vi "get Data.vi"(11 "IO in":refnum<class "IO.lvclass">) -> (3 "Data":u8 format="%02x")   [LabVIEW 2021, in "IO.lvclass"]
uses:
  IO.lvclass
  IO.lvclass/IO.ctl
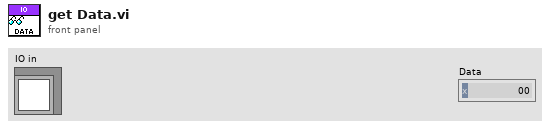
[diagram p1: front panel]
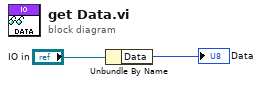
[diagram p0: block diagram]
diagram:
  n1 = Unbundle By Name("IO in") -> ("Data"=→"Data":u8)
